vi "exnSpectralBlock clear phase.vi"(1 "phase in":cluster{"f0":dbl, "df":dbl, "phase":dbl[]} {"phase" format="%.2p"; "f0" format="%0.2p"; "df" format="%0.2p"}) -> (0 "phase out":cluster{"f0":dbl, "df":dbl, "phase":dbl[]} {"phase" format="%.2p"; "f0" format="%0.2p"; "df" format="%0.2p"})   [LabVIEW 2020]
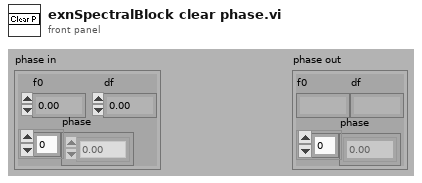
[diagram p1: front panel]
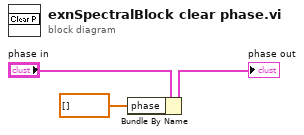
[diagram p0: block diagram]
diagram:
  n1 = Bundle By Name(cluster="phase in", "phase"=dbl[] [] ("magnitude")) -> (→"phase out":cluster{"f0":dbl, "df":dbl, "phase":dbl[]})
